vi "TCP_task_trace.vi"() -> ()   [LabVIEW 2021]
panel:
  in  "RESET MCU":bool
  in  "Keyboard":T1
  in  "stop":bool
  out "error out":errorcluster
  in  "error in (no error)":errorcluster
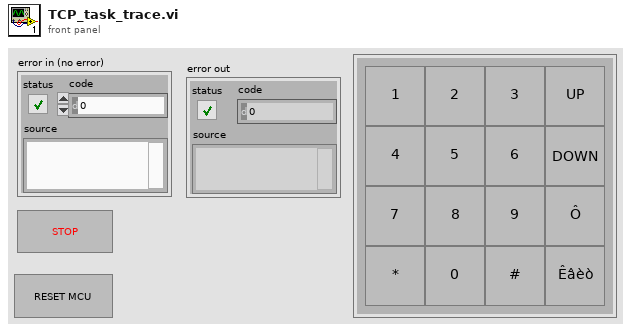
[diagram p1: front panel]
types:
  T1 = cluster{"1Btn":bool, "4Btn":bool, "7Btn":bool, "StarBtn":bool, "2Btn":bool, "5Btn":bool, "8Btn":bool, "0Btn":bool, "3Btn":bool, "6Btn":bool, "9Btn":bool, "HashBtn":bool, "UpBtn":bool, "DownBtn":bool, "FBtn":bool, "QuitBtn":bool}
  T2 = typedef "eventvkey.ctl" = enum16{"ASCII", "Enter", "Return", "Shift", "Ctrl", "Alt", "Cmd", "Opt", "Caps", "NumLock", "Clear", "Break", "Up", "Down", "Left", "Right", "Insert", "Delete", "Home", "End", "PageUp", "PageDown", "Escape", "Help", "Pause", "ScrollLock", "F1", "F2", "F3", "F4", "F5", "F6", "F7", "F8", "F9", "F10", "F11", "F12", "F13", "F14", "F15", "F16", "F17", "F18", "F19", "F20", "F21", "F22", "F23", "F24", "Play", "VolumeUp", "VolumeDown", "Mute", "Two Byte Char"}
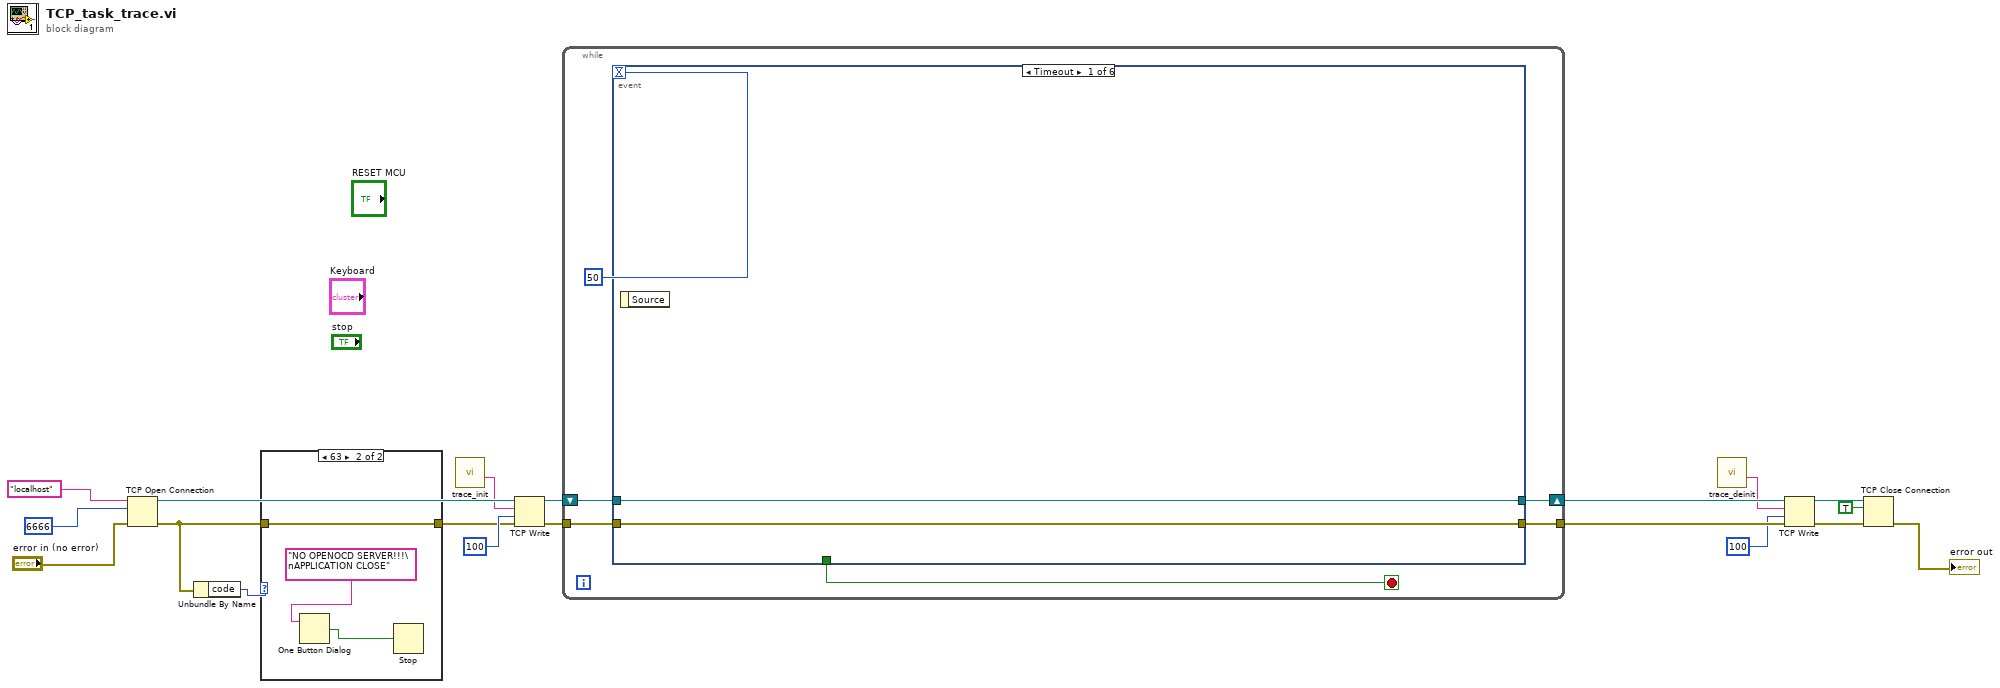
[diagram p0: block diagram]
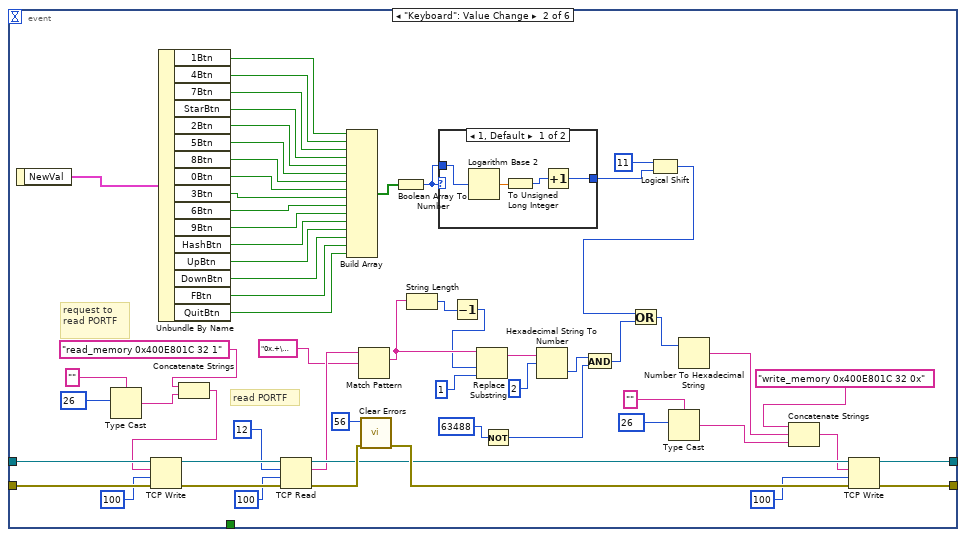
[diagram p3: hidden frame]
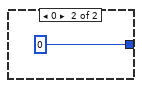
[diagram p4: hidden frame]
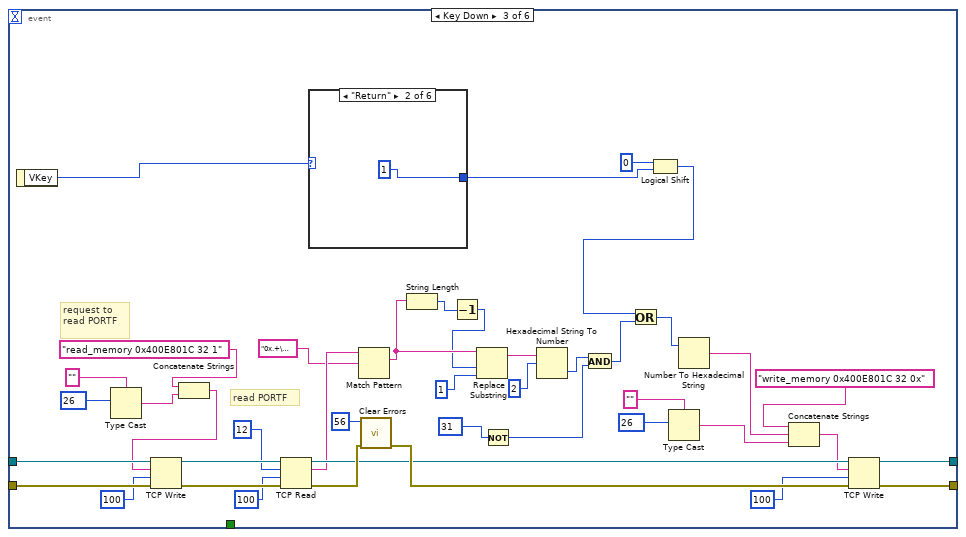
[diagram p5: hidden frame]
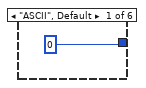
[diagram p6: hidden frame]
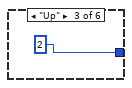
[diagram p7: hidden frame]
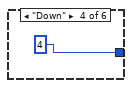
[diagram p8: hidden frame]
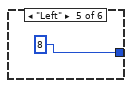
[diagram p9: hidden frame]
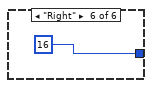
[diagram p10: hidden frame]
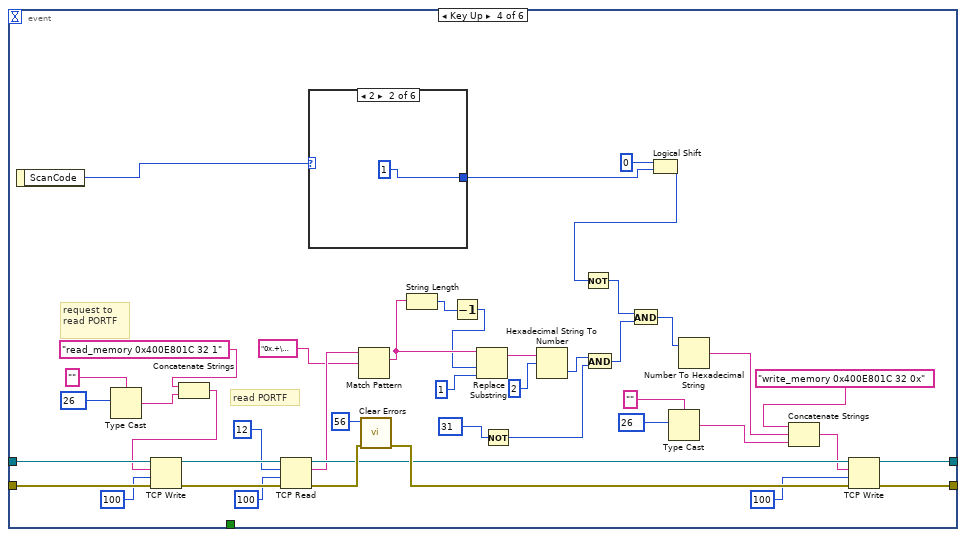
[diagram p11: hidden frame]
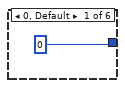
[diagram p12: hidden frame]
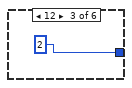
[diagram p13: hidden frame]
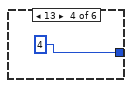
[diagram p14: hidden frame]
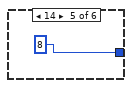
[diagram p15: hidden frame]
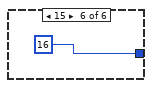
[diagram p16: hidden frame]
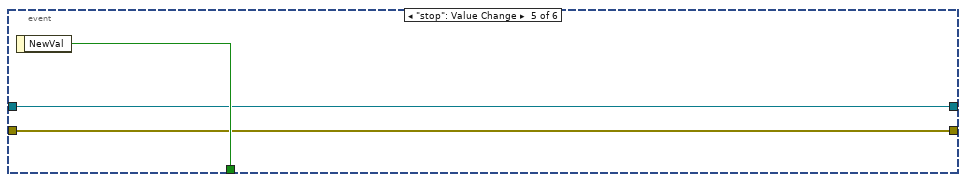
[diagram p17: hidden frame]
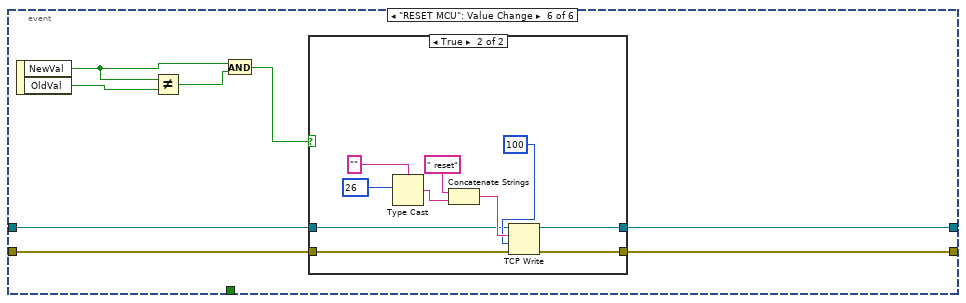
[diagram p18: hidden frame]
diagram:
  n1 = TCP Open Connection(address="localhost", remote port or service name=u16 6666 ("local port (0)"), error in (no error)="error in (no error)") -> (connection ID=w14:refnum<k5>, error out=w2:errorcluster)  [unwired: 2 in]
  n2 = Unbundle By Name(w2) -> ("code"=w3:i32)
  n3 = case shown="63" w3 {
    tunnel: w2 -> [w20 w21]
    tunnel: [w20 w21] -> w1
    frame 0, Default {
    }
    frame 63 {
      n4 = One Button Dialog(message="NO OPENOCD SERVER!!!\nAPPLICATION CLOSE") -> (true=w22:bool)  [unwired: 1 in]
      n5 = Stop(stop? (T)=w22) -> ()
    }
  }
  n6 = call "trace_init.vi"() -> ("Init seq."=w11:string)  [unwired: 11 in]
  n7 = TCP Write(connection ID=w14, data in=w11, error in (no error)=w1, 9:100 ("timeout ms (25000)")) -> (connection ID out=w13:refnum<k5>, error out=w12:errorcluster)  [unwired: 1 out]
  n8 = while {
    tunnel: w12 -> [w26]
    tunnel: [w24] -> w9
    shift-right: [w25] -> w10
    shift-left: w13 -> [w27]
    stop <- w28 stop-if-true
    n9 = event shown="[0] Timeout" {
      selector: _ -> [_ _ _ _ _ _]
      dyn-events: _ -> [_ _ _ _ _ _]
      timeout: 50 -> [_ _ _ _ _ _]
      tunnel: [_ _ _ _ w196 _] -> w28
      tunnel: w27 -> [w31 w91 w138 w187 w195 w204]
      tunnel: w26 -> [w30 w90 w137 w186 w194 w202]
      tunnel: [w31 w54 w121 w171 w195 w203] -> w25
      tunnel: [w30 w53 w120 w170 w194 w201] -> w24
      event Timeout {
        n10 = event-data() -> ()  [unwired: 1 in, 1 out]
      }
      event "Keyboard": Value Change {
        # "read PORTF"
        # "request to\nread PORTF"
        n11 = event-data() -> ("NewVal"=w77:T1)  [unwired: 1 in]
        n12 = Type Cast(type="", x=u8 26) -> (*(type *) &x=w79:string)
        n13 = Unbundle By Name(w77) -> ("1Btn"=w76:bool, "4Btn"=w75:bool, "7Btn"=w74:bool, "StarBtn"=w73:bool, "2Btn"=w72:bool, "5Btn"=w71:bool, "8Btn"=w70:bool, "0Btn"=w69:bool, "3Btn"=w68:bool, "6Btn"=w67:bool, "9Btn"=w66:bool, "HashBtn"=w65:bool, "UpBtn"=w64:bool, "DownBtn"=w63:bool, "FBtn"=w62:bool, "QuitBtn"=w61:bool)
        n14 = Concatenate Strings("read_memory 0x400E801C 32 1" ("data in"), w79) -> (w78:string)
        n15 = TCP Write(connection ID=w91, data in=w78, error in (no error)=w90, 9:100 ("timeout ms (25000)")) -> (connection ID out=w86:refnum<k5>, error out=w87:errorcluster)  [unwired: 1 out]
        n16 = TCP Read(connection ID=w86, bytes to read=12, error in (no error)=w87, 9:100 ("timeout ms (25000)")) -> (connection ID out=w51:refnum<k5>, data out=w44:string, error out=w85:errorcluster)  [unwired: 1 in]
        n17 = Build Array(w76, w75, w74, w73, w72, w71, w70, w69, w68, w67, w66, w65, w64, w63, w62, w61) -> (w60:bool[])
        n18 = Match Pattern(string=w44, regular expression="0x.+\u001a") -> (match substring=w41:string)  [unwired: 1 in, 3 out]
        n19 = call <vilib>:"Clear Errors.vi"("error in (no error)"=w85, "specific error code to clear (0: all)"=56) -> ("error out"=w52:errorcluster)  [unwired: 4 in, 1 out]
        n20 = Boolean Array To Number(Boolean array=w60) -> (number=w59:u32)
        n21 = String Length(string=w41) -> (length=w42:i32)
        n22 = case shown="1, Default" w59 {
          tunnel: w59 -> [w93 _]
          tunnel: [w92 0] -> w58
          frame 1, Default {
            n23 = Logarithm Base 2(1:w93) -> (0:w94:dbl)
            n24 = To Unsigned Long Integer(number=w94) -> (unsigned 32bit integer=w95:u32)
            n25 = Increment(x=w95) -> (x+1=w92:u32)
          }
          frame 0 {
          }
        }
        n26 = Decrement(x=w42) -> (x-1=w40:i32)
        n27 = Replace Substring(2:1 ("length (len. of substring)"), 3:w40, 5:w41) -> (1:w38:string)  [unwired: 1 in, 1 out]
        n28 = Not(x=u32 63488) -> (.not. x?=w45:u32)
        n29 = Hexadecimal String To Number(string=w38, offset=2) -> (number=w36:u32)  [unwired: 1 in, 1 out]
        n30 = And(x=w36, y=w45) -> (x .and. y?=w35:u32)
        n31 = Logical Shift(y=i16 11, x=w58) -> (x << y=w55:u32)
        n32 = Or(x=w55, y=w35) -> (x .or. y?=w34:u32)
        n33 = Type Cast(type="", x=u8 26) -> (*(type *) &x=w46:string)
        n34 = Number To Hexadecimal String(2:w34) -> (0:w33:string)  [unwired: 1 in]
        n35 = Concatenate Strings("write_memory 0x400E801C 32 0x", w33, w46) -> (w32:string)
        n36 = TCP Write(connection ID=w51, data in=w32, error in (no error)=w52, 9:100 ("timeout ms (25000)")) -> (connection ID out=w54:refnum<k5>, error out=w53:errorcluster)  [unwired: 1 out]
      }
      event Key Down {
        # "read PORTF"
        # "request to\nread PORTF"
        n37 = event-data() -> ("VKey"=w98:T2)  [unwired: 1 in]
        n38 = Type Cast(type="", x=u8 26) -> (*(type *) &x=w126:string)
        n39 = Concatenate Strings("read_memory 0x400E801C 32 1" ("data in"), w126) -> (w125:string)
        n40 = TCP Write(connection ID=w138, data in=w125, error in (no error)=w137, 9:100 ("timeout ms (25000)")) -> (connection ID out=w133:refnum<k5>, error out=w134:errorcluster)  [unwired: 1 out]
        n41 = TCP Read(connection ID=w133, bytes to read=12, error in (no error)=w134, 9:100 ("timeout ms (25000)")) -> (connection ID out=w118:refnum<k5>, data out=w111:string, error out=w132:errorcluster)  [unwired: 1 in]
        n42 = case shown="\"Return\"" w98 {
          tunnel: [u32 0 u32 1 u32 2 u32 4 u32 8 u32 16] -> w97
          frame "ASCII", Default {
          }
          frame "Return" {
          }
          frame "Up" {
          }
          frame "Down" {
          }
          frame "Left" {
          }
          frame "Right" {
          }
        }
        n43 = Match Pattern(string=w111, regular expression="0x.+\u001a") -> (match substring=w108:string)  [unwired: 1 in, 3 out]
        n44 = call <vilib>:"Clear Errors.vi"("error in (no error)"=w132, "specific error code to clear (0: all)"=56) -> ("error out"=w119:errorcluster)  [unwired: 4 in, 1 out]
        n45 = String Length(string=w108) -> (length=w109:i32)
        n46 = Decrement(x=w109) -> (x-1=w107:i32)
        n47 = Replace Substring(2:1 ("length (len. of substring)"), 3:w107, 5:w108) -> (1:w105:string)  [unwired: 1 in, 1 out]
        n48 = Not(x=u32 31) -> (.not. x?=w112:u32)
        n49 = Hexadecimal String To Number(string=w105, offset=2) -> (number=w103:u32)  [unwired: 1 in, 1 out]
        n50 = And(x=w103, y=w112) -> (x .and. y?=w102:u32)
        n51 = Logical Shift(y=i16 0, x=w97) -> (x << y=w122:u32)
        n52 = Or(x=w122, y=w102) -> (x .or. y?=w101:u32)
        n53 = Type Cast(type="", x=u8 26) -> (*(type *) &x=w113:string)
        n54 = Number To Hexadecimal String(2:w101) -> (0:w100:string)  [unwired: 1 in]
        n55 = Concatenate Strings("write_memory 0x400E801C 32 0x", w100, w113) -> (w99:string)
        n56 = TCP Write(connection ID=w118, data in=w99, error in (no error)=w119, 9:100 ("timeout ms (25000)")) -> (connection ID out=w121:refnum<k5>, error out=w120:errorcluster)  [unwired: 1 out]
      }
      event Key Up {
        # "read PORTF"
        # "request to\nread PORTF"
        n57 = event-data() -> ("ScanCode"=w148:i16)  [unwired: 1 in]
        n58 = Type Cast(type="", x=u8 26) -> (*(type *) &x=w175:string)
        n59 = Concatenate Strings("read_memory 0x400E801C 32 1" ("data in"), w175) -> (w174:string)
        n60 = TCP Write(connection ID=w187, data in=w174, error in (no error)=w186, 9:100 ("timeout ms (25000)")) -> (connection ID out=w182:refnum<k5>, error out=w183:errorcluster)  [unwired: 1 out]
        n61 = TCP Read(connection ID=w182, bytes to read=12, error in (no error)=w183, 9:100 ("timeout ms (25000)")) -> (connection ID out=w168:refnum<k5>, data out=w161:string, error out=w181:errorcluster)  [unwired: 1 in]
        n62 = case shown="2" w148 {
          tunnel: [u32 0 u32 1 u32 2 u32 4 u32 8 u32 16] -> w147
          frame 0, Default {
          }
          frame 2 {
          }
          frame 12 {
          }
          frame 13 {
          }
          frame 14 {
          }
          frame 15 {
          }
        }
        n63 = Match Pattern(string=w161, regular expression="0x.+\u001a") -> (match substring=w158:string)  [unwired: 1 in, 3 out]
        n64 = call <vilib>:"Clear Errors.vi"("error in (no error)"=w181, "specific error code to clear (0: all)"=56) -> ("error out"=w169:errorcluster)  [unwired: 4 in, 1 out]
        n65 = String Length(string=w158) -> (length=w159:i32)
        n66 = Decrement(x=w159) -> (x-1=w157:i32)
        n67 = Replace Substring(2:1 ("length (len. of substring)"), 3:w157, 5:w158) -> (1:w155:string)  [unwired: 1 in, 1 out]
        n68 = Not(x=u32 31) -> (.not. x?=w162:u32)
        n69 = Hexadecimal String To Number(string=w155, offset=2) -> (number=w153:u32)  [unwired: 1 in, 1 out]
        n70 = And(x=w153, y=w162) -> (x .and. y?=w152:u32)
        n71 = Logical Shift(y=i16 0, x=w147) -> (x << y=w146:u32)
        n72 = Not(x=w146) -> (.not. x?=w145:u32)
        n73 = And(x=w145, y=w152) -> (x .and. y?=w151:u32)
        n74 = Type Cast(type="", x=u8 26) -> (*(type *) &x=w163:string)
        n75 = Number To Hexadecimal String(2:w151) -> (0:w150:string)  [unwired: 1 in]
        n76 = Concatenate Strings("write_memory 0x400E801C 32 0x", w150, w163) -> (w149:string)
        n77 = TCP Write(connection ID=w168, data in=w149, error in (no error)=w169, 9:100 ("timeout ms (25000)")) -> (connection ID out=w171:refnum<k5>, error out=w170:errorcluster)  [unwired: 1 out]
      }
      event "stop": Value Change {
        n78 = event-data() -> ("NewVal"=w196:bool)  [unwired: 1 in]
      }
      event "RESET MCU": Value Change {
        n79 = event-data() -> ("NewVal"=w198:bool, "OldVal"=w200:bool)  [unwired: 1 in]
        n80 = Not Equal?(x=w198, y=w200) -> (x != y?=w199:bool)
        n81 = And(x=w198, y=w199) -> (x .and. y?=w197:bool)
        n82 = case shown="True" w197 {
          tunnel: w204 -> [w206 w210]
          tunnel: [w206 w209] -> w203
          tunnel: w202 -> [w205 w208]
          tunnel: [w205 w207] -> w201
          frame False {
          }
          frame True {
            n83 = Type Cast(type="", x=u8 26) -> (*(type *) &x=w216:string)
            n84 = Concatenate Strings(" reset", w216) -> (w215:string)
            n85 = TCP Write(connection ID=w210, data in=w215, error in (no error)=w208, 9:100 ("timeout ms (25000)")) -> (connection ID out=w209:refnum<k5>, error out=w207:errorcluster)  [unwired: 1 out]
          }
        }
      }
    }
  }
  n86 = call "trace_deinit.vi"() -> ("deInit seq."=w8:string)  [unwired: 11 in]
  n87 = TCP Write(connection ID=w10, data in=w8, error in (no error)=w9, 9:100 ("timeout ms (25000)")) -> (connection ID out=w6:refnum<k5>, error out=w5:errorcluster)  [unwired: 1 out]
  n88 = TCP Close Connection(connection ID=w6, abort (F)=TRUE, error in (no error)=w5) -> (error out=→"error out":errorcluster)  [unwired: 1 out]
